vi "Aggregated var speed Test.vi"() -> ()   [LabVIEW 2021]
uses:
  <vilib>/TSA/Abstract Data Classes/Abs_Types/Double Float/Support/Type.ctl
  Source/Omni-Bus/Omni_Bus.lvclass
  Source/Omni-Bus/Support/Broad Types.ctl
  <vilib>/TSA/Abstract Data Classes/Abs_Types/Type/Abs_Type.lvclass
  <vilib>/TSA/Abstract Data Classes/Abs_Types/Type/Abs_Type.lvclass/Abs_Type.ctl
  Source/Omni-Bus/Omni_Bus.lvclass/Omni_Bus.ctl
  Source/Omni-Bus/Support/FindVar.vi
  <vilib>/Utility/error.llb/Clear Errors.vi
  Source/Omni-Bus/Properties/Read Var Map.vi
  <vilib>/TSA/Abstract Data Classes/Abs_Types/Type/Properties/Read Tag.vi
  <vilib>/TSA/Abstract Data Classes/Abs_Types/Boolean/Abs_Boolean.lvclass
  C:/Program Files (x86)/National Instruments/LabVIEW 2021/vi.lib/TSA/Abstract Data Classes/Abs_Types/Type/Abs_Type.lvclass
  <vilib>/TSA/Abstract Data Classes/Constants/Support/DBL/Const_DBL.lvclass
  <vilib>/TSA/Abstract Data Classes/Abs_Types/String/Abs_String.lvclass
  <vilib>/TSA/Abstract Data Classes/Abs_Types/I32 Integer/Abs_I32 Integer.lvclass
  Source/Aggregator Bus/Aggregator Bus.lvclass
  C:/Users/Tim/Documents/GitHub/Omni-Bus/Source/Omni-Bus/Bus Access/Bus_Access.lvclass
  <vilib>/TSA/Abstract Data Classes/Abs_Types/Double Float/Abs_Double Float.lvclass
  <vilib>/TSA/Abstract Data Classes/Abs_Types/Value/Abs_Value.lvclass
  <vilib>/TSA/Abstract Data Classes/Constants/Support/Bool/Bool.vi
  <vilib>/TSA/Abstract Data Classes/Constants/Support/DBL/DBL.vi
  <vilib>/TSA/Abstract Data Classes/Constants/Support/Str/Str.vi
  <vilib>/TSA/Abstract Data Classes/Constants/Support/I32/I32.vi
  Source/Omni-Bus/Support/Check For Read Only Error.vi
  Source/Omni-Bus/Support/Incorrect Tag String Error.vi
  <vilib>/TSA/Abstract Data Classes/Constants/Support/Str/Const_Str.lvclass
  <vilib>/TSA/Abstract Data Classes/Constants/Support/Bool/Const_Bool.lvclass
  <vilib>/TSA/Abstract Data Classes/Constants/Support/I32/Const_I32.lvclass
panel:
  out "error out":errorcluster
  out "x-y":dbl
  out "Value":T1
  out "Tags":string[](array[string])
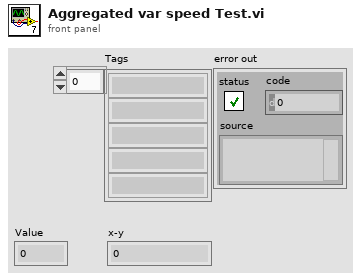
[diagram p1: front panel]
types:
  T1 = typedef "Abs_Double Float.lvclass/Type.ctl" = dbl
  T2 = typedef "Omni_Bus.lvclass/Broad Types.ctl" = enum16{"All Tags", "NI Specific Type", "Boolean", "String", "Numeric", "Float", "Integer", "Collection", "All Value Types", "Non Value Types"}
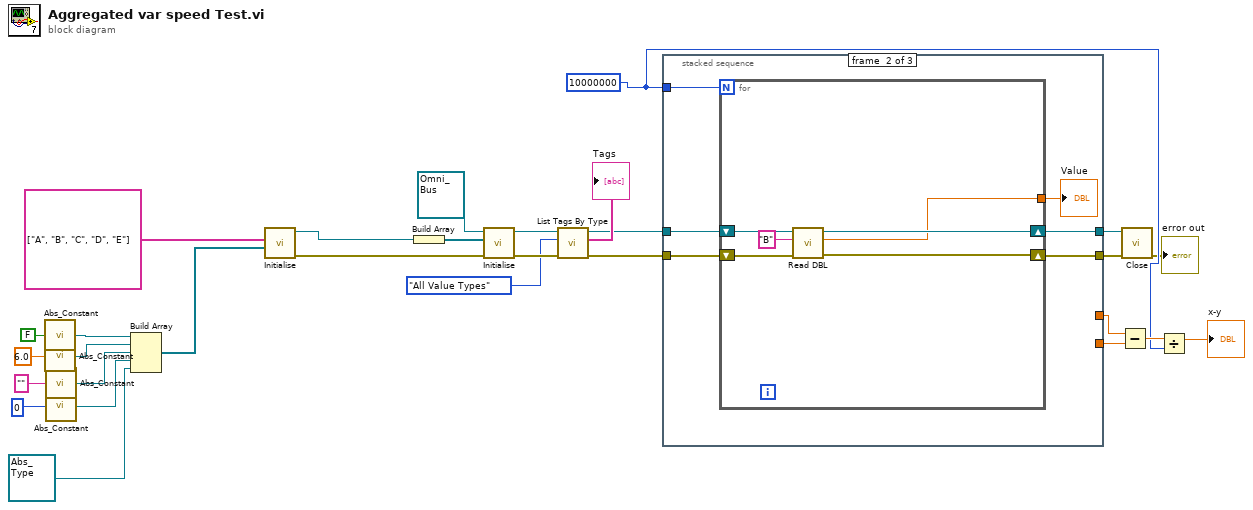
[diagram p0: block diagram]
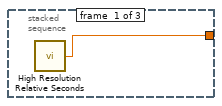
[diagram p2: hidden frame]
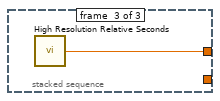
[diagram p3: hidden frame]
diagram:
  w7 = 10000000
  n1 = call-poly <vilib>:"Abs_Constant.vi"("Boolean"=FALSE) -> ("Abs_Boolean.lvclass"=w27:refnum<class "Abs_Boolean.lvclass">)  [unwired: 4 in]
  n2 = call-poly <vilib>:"Abs_Constant.vi"("Value"=6.0) -> ("Constant"=w26:refnum<class "Const_DBL.lvclass">)  [unwired: 4 in]
  n3 = call-poly <vilib>:"Abs_Constant.vi"("String"="") -> ("Abs_String.lvclass"=w25:refnum<class "Abs_String.lvclass">)  [unwired: 4 in]
  n4 = call-poly <vilib>:"Abs_Constant.vi"("Value"=0) -> ("Constant"=w18:refnum<class "Abs_I32 Integer.lvclass">)  [unwired: 4 in]
  n5 = Build Array(w27, w26, w25, w18, refnum<class "Abs_Type.lvclass"> refnum ("Abs_Type.lvclass")) -> (w1:refnum<class "Abs_Type.lvclass">[])
  n6 = call "Initialise.vi"("Values"=w1, "Tags"=string[] ["A", "B", "C", "D", "E"]) -> ("error out"=w4:errorcluster, "Aggregator Bus out"=w3:refnum<class "Aggregator Bus.lvclass">)  [unwired: 8 in]
  n7 = Build Array(w3) -> (w28:refnum<class "Aggregator Bus.lvclass">[])
  n8 = call-dynamic "Initialise.vi"("error in (no error)"=w4, "Bus Access"=w28, "Var Bus in"=refnum<class "Omni_Bus.lvclass"> refnum) -> ("error out"=w21:errorcluster, "Var Bus out"=w22:refnum<class "Omni_Bus.lvclass">)  [unwired: 7 in]
  n9 = call "List Tags By Type.vi"("error in (no error)"=w21, "Broad Types"=Broad_Types."All Value Types", "Var Bus in"=w22) -> ("error out"=w14:errorcluster, "Tags"=→"Tags":string[], "Var Bus out"=w15:refnum<class "Omni_Bus.lvclass">)  [unwired: 5 in, 1 out]
  n10 = stacked-sequence {
    tunnel: w15 -> [_ w36 _]
    tunnel: w14 -> [_ w35 _]
    tunnel: [_ w34 _] -> w13
    tunnel: [_ w33 _] -> w12
    tunnel: [_ _ w43] -> w11
    tunnel: [w30 _ _] -> w10
    tunnel: w7 -> [_ w31 _]
    frame #0 {
      n11 = call <vilib>:"High Resolution Relative Seconds.vi"() -> ("relative seconds"=w30:dbl)
    }
    frame #1 {
      n12 = for {
        N: w31 -> [_]
        shift-right: [w41] -> w34
        shift-left: w36 -> [w42]
        shift-right: [w39] -> w33
        shift-left: w35 -> [w40]
        tunnel: [w38] -> w32
        n13 = call "Read DBL.vi"("error in (no error)"=w40, "Tag"="B", "Var Bus in"=w42) -> ("error out"=w39:errorcluster, "Numeric"=w38:dbl, "Var Bus out"=w41:refnum<class "Omni_Bus.lvclass">)  [unwired: 6 in]
      }
      "Value" <- w32
    }
    frame #2 {
      n14 = call <vilib>:"High Resolution Relative Seconds.vi"() -> ("relative seconds"=w43:dbl)
    }
  }
  n15 = Subtract(x=w11, y=w10) -> (x-y=w9:dbl)
  n16 = call-dynamic "Close.vi"("error in (no error)"=w12, "Data in"=w13) -> ("error out"=→"error out":errorcluster)  [unwired: 8 in, 1 out]
  n17 = Divide(x=w9, y=w7) -> (x/y=→"x-y":dbl)
